vi "powermeter-close.vi"(2 "error in (no error)":errorcluster, 3 "VISA resource name":refnum<visa-resource-name>) -> (0 "error out":errorcluster)   [LabVIEW 2015]
doc: "Closes the VISA session\nSets the connected instrument in local mode (default option)"
uses:
  <vilib>/Instr/_visa.llb/VISA GPIB Control REN Mode.ctl
panel:
  in  "Mode":T1=2 items=["Deassert REN", "Assert REN", "Go To Local; Deassert REN ", "Assert REN; Address Device", "Local Lockout (Addressed Devices)", "Local Lockout (This Device)", "Go To Local"]
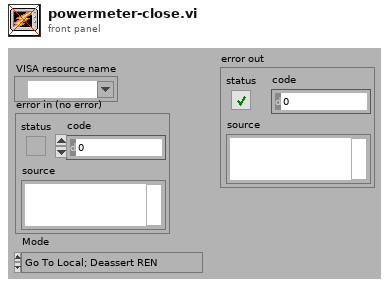
[diagram p1: front panel]
types:
  T1 = typedef "VISA GPIB Control REN Mode.ctl" = u16
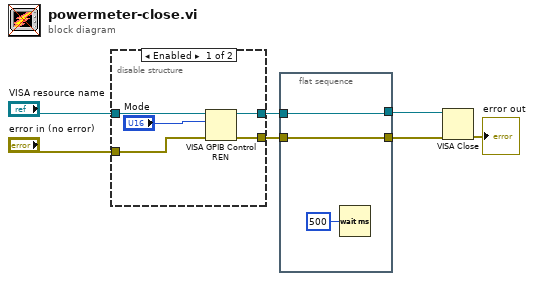
[diagram p0: block diagram]
diagram:
  n1 = disable-structure shown="Enabled" {
    disable-tunnel: "VISA resource name" -> [w11 _]
    disable-tunnel: "error in (no error)" -> [w10 _]
    disable-tunnel: [w9 _] -> w5
    disable-tunnel: [w8 _] -> w3
    frame Enabled {
      n2 = VISA GPIB Control REN(8:w10, 10:"Mode", 11:w11) -> (0:w8:errorcluster, 3:w9:refnum<visa-resource-name>)
    }
    frame Disabled {
    }
  }
  n3 = flat-sequence {
    tunnel: [w15] -> w4
    tunnel: w5 -> [w15]
    tunnel: w3 -> [w14]
    tunnel: [w14] -> w2
    frame #0 {
      n4 = Wait (ms)(milliseconds to wait=u32 500) -> ()  [unwired: 1 out]
    }
  }
  n5 = VISA Close(VISA resource name=w4, error in (no error)=w2) -> (error out=→"error out":errorcluster)
